vi "Test Test Finder Find Dynamic Test Methods in Test Case Class.vi"(8 "error in (no error)":errorcluster, 11 "Test Finder In":refnum<class "Test Finder Test.lvclass">) -> (0 "error out":errorcluster, 3 "Test Finder Out":refnum<class "Test Finder Test.lvclass">)   [LabVIEW 2020, in "LUnit Tests.lvlib" / "Test Finder Test.lvclass"]
uses:
  Test Finder Test.lvclass
  C:/Program Files (x86)/National Instruments/LabVIEW 2020/vi.lib/Astemes/LUnit/Test Case.lvclass
  Test Dummys/Descending Test Test Case/Descending Test Test Case.lvclass
  Test Finder Test.lvclass/Test Finder Test.ctl
  <vilib>/Astemes/LUnit/Test Case.lvclass/Test Case.ctl
  <vilib>/Astemes/LUnit/LUnit Assertion Result.lvclass/LUnit Assertion Result.ctl
  <vilib>/Astemes/LUnit/LUnit Test Case Result.lvclass/LUnit Test Case Result.ctl
  <vilib>/Astemes/LUnit/LUnit Method Result.lvclass/LUnit Method Result.ctl
  48b63480-a817-4be7-af3b-75100f58d784.vi
  <vilib>/Astemes/LUnit/Palette/Pass.vi
  <vilib>/Astemes/LUnit/Palette/Fail.vi
  <vilib>/Astemes/LUnit/Compare Variants.vi
  <vilib>/Astemes/LUnit/Describe Comparison.vi
  <vilib>/Astemes/LUnit/Set Assertion Type.vi
  <vilib>/Astemes/LUnit/Add test result.vi
  <vilib>/Astemes/LUnit/LUnit Write Passed.vi
  <vilib>/Astemes/LUnit/LUnit Write Message.vi
  <vilib>/Astemes/LUnit/LUnit Write Description.vi
  <vilib>/Astemes/LUnit/Variant to string.vi
  <vilib>/Astemes/LUnit/LUnit Write Assertion Type.vi
  <vilib>/Astemes/LUnit/LUnit Record Assertion Result.vi
  <vilib>/Astemes/LUnit/LUnit Aggregate Assertion Results.vi
  <vilib>/Astemes/LUnit/Assertion Result/LUnit Read Status.vi
  <vilib>/Astemes/LUnit/LUnit Read Message.vi
  <vilib>/Astemes/LUnit/LUnit Read Description.vi
  <vilib>/Astemes/LUnit/Method Result/LUnit Merge Status.vi
  <vilib>/Astemes/LUnit/LUnit Concatenate result strings.vi
  <vilib>/Utility/Data Type/Get Type Information.vi
  <vilib>/Utility/LVClass/Get LV Class Name.vi
  source/Framework/Helper Classes/Test Finder/Test Finder.lvclass
  <vilib>/Astemes/LUnit/LUnit Assertion Result.lvclass
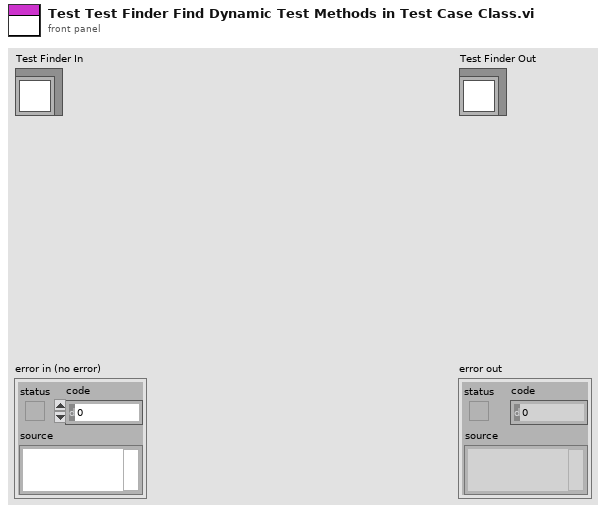
[diagram p1: front panel]
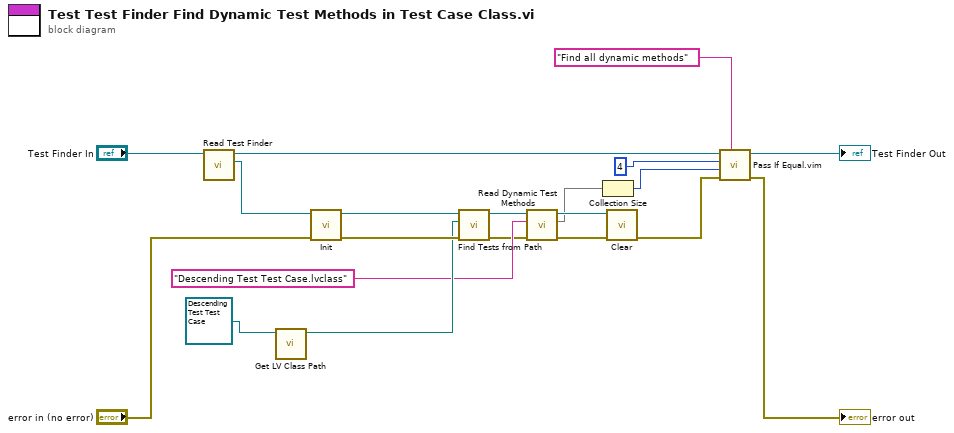
[diagram p0: block diagram]
diagram:
  n1 = call "Read Test Finder.vi"("Test Finder In"="Test Finder In") -> ("Test Finder.lvclass"=w19:refnum<class "Test Finder.lvclass">, "Test Finder Out"=w8:refnum<class "Test Finder Test.lvclass">)  [unwired: 8 in, 1 out]
  n2 = call <vilib>:"Get LV Class Path.vi"("object"=refnum<class "Descending Test Test Case.lvclass"> refnum ("Descending Test Test Case.lvclass")) -> ("class path"=w15:path)  [unwired: 9 in, 1 out]
  n3 = call-dynamic "Init.vi"("error in (no error)"="error in (no error)", "Test Finder in"=w19) -> ("error out"=w17:errorcluster, "Test Finder out"=w18:refnum<class "Test Finder.lvclass">)  [unwired: 8 in]
  n4 = call-dynamic "Find Tests from Path.vi"("error in (no error)"=w17, "Project or Class Path"=w15, "Test Case Finder In"=w18) -> ("error out"=w11:errorcluster, "Test Case Finder Out"=w13:refnum<class "Test Finder.lvclass">)  [unwired: 7 in]
  n5 = call "Read Dynamic Test Methods.vi"("error in (no error)"=w11, "Test Case"="Descending Test Test Case.lvclass", "Test Case Finder In"=w13) -> ("error out"=w10:errorcluster, "Dynamic Test Methods"=w3:map{string, path}, "Test Case Finder Out"=w12:refnum<class "Test Finder.lvclass">)  [unwired: 6 in]
  n6 = Collection Size(1:w3) -> (0:w2:i32)
  n7 = call "Clear.vi"("error in (no error)"=w10, "Test Finder in"=w12) -> ("error out"=w6:errorcluster)  [unwired: 8 in, 1 out]
  n8 = call "Pass If Equal.vim"("Description"="Find all dynamic methods", "error in (no error)"=w6, "Actual"=w2, "Expected"=4 ("size"), "LUnit Test Case In"=w8) -> ("error out"=→"error out":errorcluster, "LUnit Test Case Out"=→"Test Finder Out":refnum<class "Test Finder Test.lvclass">)  [unwired: 5 in]
